vi "Get Reset ID.vi"(2 "Function":enum16{"Get ID", "Reset ID"}(ring)) -> (8 "ID":string)   [LabVIEW 2020]
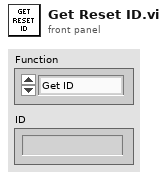
[diagram p1: front panel]
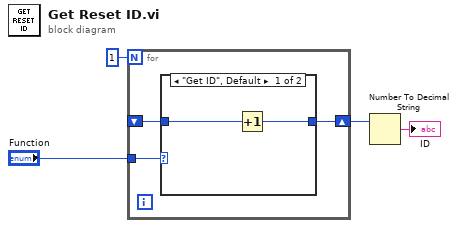
[diagram p0: block diagram]
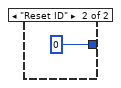
[diagram p2: hidden frame]
diagram:
  n1 = for {
    N: 1 -> [_]
    tunnel: "Function" -> [w7]
    shift-right: [w6] -> w3
    shift-left: _ -> [w5]
    n2 = case shown="\"Get ID\", Default" w7 {
      tunnel: [w8 0] -> w6
      tunnel: w5 -> [w9 _]
      frame "Get ID", Default {
        n3 = Increment(x=w9) -> (x+1=w8:i32)
      }
      frame "Reset ID" {
      }
    }
  }
  n4 = Number To Decimal String(number=w3) -> (decimal integer string=→"ID":string)  [unwired: 1 in]
